vi "CalculateTargetRange.vi"(0 "object in":refnum<class "ShootTactic_v2.lvclass">, 5 "error in (no error)":errorcluster) -> (14 "object out":refnum<class "ShootTactic_v2.lvclass">, 19 "error out":errorcluster)   [LabVIEW 2023, in "ShootTactic_v2.lvclass"]
uses:
  ShootTactic_v2.lvclass
  KickTactic_class/KickTactic.lvclass
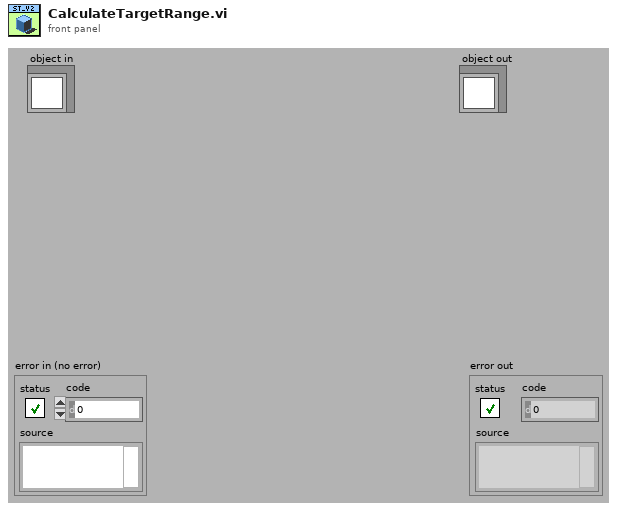
[diagram p1: front panel]
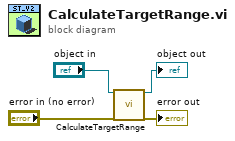
[diagram p0: block diagram]
diagram:
  n1 = call-parent "CalculateTargetRange.vi"("object in"="object in", "error in (no error)"="error in (no error)") -> ("object out"=→"object out":refnum<class "ShootTactic_v2.lvclass">, "error out"=→"error out":errorcluster)  [unwired: 16 in]
